vi "GFITS_LibGetRoi.vi"(8 "error in (no error)":errorcluster) -> (0 "error IO":errorcluster, 3 "roi?":bool, 4 "ylen":u32, 5 "ystart out":u32, 6 "xlen out":u32, 7 "xstart out":u32)   [LabVIEW 2016]
uses:
  c/lib/libgfits.so
panel:
  in  "ylen":u32
  in  "xlen":u32
  in  "ystart":u32
  in  "xstart":u32
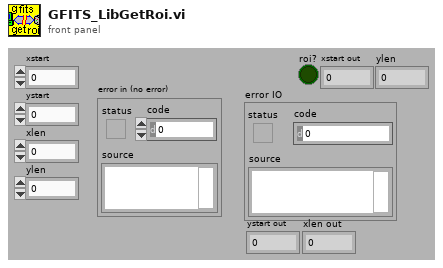
[diagram p1: front panel]
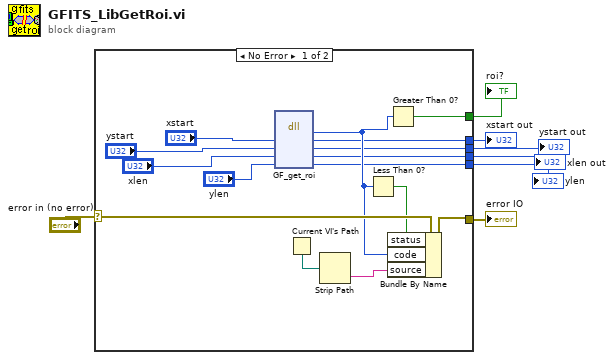
[diagram p0: block diagram]
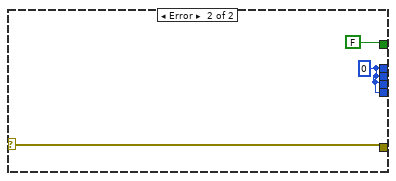
[diagram p2: hidden frame]
diagram:
  n1 = case shown="No Error" "error in (no error)" {
    selector: "error in (no error)" -> [w22 w25]
    tunnel: [w18 w25] -> w6
    tunnel: [w12 FALSE] -> w5
    tunnel: [w11 w23] -> w4
    tunnel: [w10 w23] -> w3
    tunnel: [w9 w23] -> w2
    tunnel: [w8 w23] -> w1
    frame No Error {
      n2 = dll-call lib="home/simager/panview/PAN/Modules/GFITS/private/c/lib/libgfits.so" fn="GF_get_roi"("xstart"="xstart", "ystart"="ystart", "xlen"="xlen", "ylen"="ylen") -> ("return type"=w13:i32, "xstart"=w11:u32, "ystart"=w10:u32, "xlen"=w9:u32, "ylen"=w8:u32)  [unwired: 3 in, 2 out]
      n3 = Current VI's Path() -> (path=w20:path)
      n4 = Strip Path(path=w20) -> (name=w19:string)  [unwired: 1 out]
      n5 = Less Than 0?(x=w13) -> (x < 0?=w21:bool)
      n6 = Greater Than 0?(x=w13) -> (x > 0?=w12:bool)
      n7 = Bundle By Name(cluster=w22, "status"=w21, "code"=w13, "source"=w19) -> (w18:errorcluster)
    }
    frame Error {
      w23 = u32 0 ("xstart")
    }
  }
  "error IO" <- w6
  "roi?" <- w5
  "xstart out" <- w4
  "ystart out" <- w3
  "xlen out" <- w2
  "ylen" <- w1
